vi "Breakdown Analysis Report.vi"(8 "error in (no error)":errorcluster) -> ()   [LabVIEW 2017]
uses:
  <vilib>/Utility/miscctls.llb/LVRowAndColumnTypeDef.ctl
  <vilib>/addons/database/Connection.llb/DB Tools Open Connec (Path).vi
  <vilib>/Utility/file.llb/Write Delimited Spreadsheet (string).vi
  <vilib>/addons/database/NI_Database_API.lvlib
panel:
  in  "Back 2":bool
  in  "Download 2":bool
  in  "Get Rport":bool
  out "index of element":i32
  out "Array":string[][](array[string])
  in  "(X,Y)":string
  out "subarray":string[](array[string])
  in  "Export to Excel":bool
  in  "Shift":string(combo)
  out "error out":errorcluster
  in  "Tab Control":enum32{"Statistical", "Graphical"}(tab)
  out "Table":string[][](table)
  out "Run-Time Status":cluster{dbl[], dbl[]}(graph)
  in  "Select Line":string(combo)
  in  "To Date":timestamp format="%<%Y-%m-%d>T"
  in  "Form Date":timestamp format="%<%Y-%m-%d>T"
  in  "Delete":bool
  in  "Edit":bool
  in  "Select Stakeholder":string(combo)
  in  "Get Report":bool
  # "Breakdown Analysis Report"
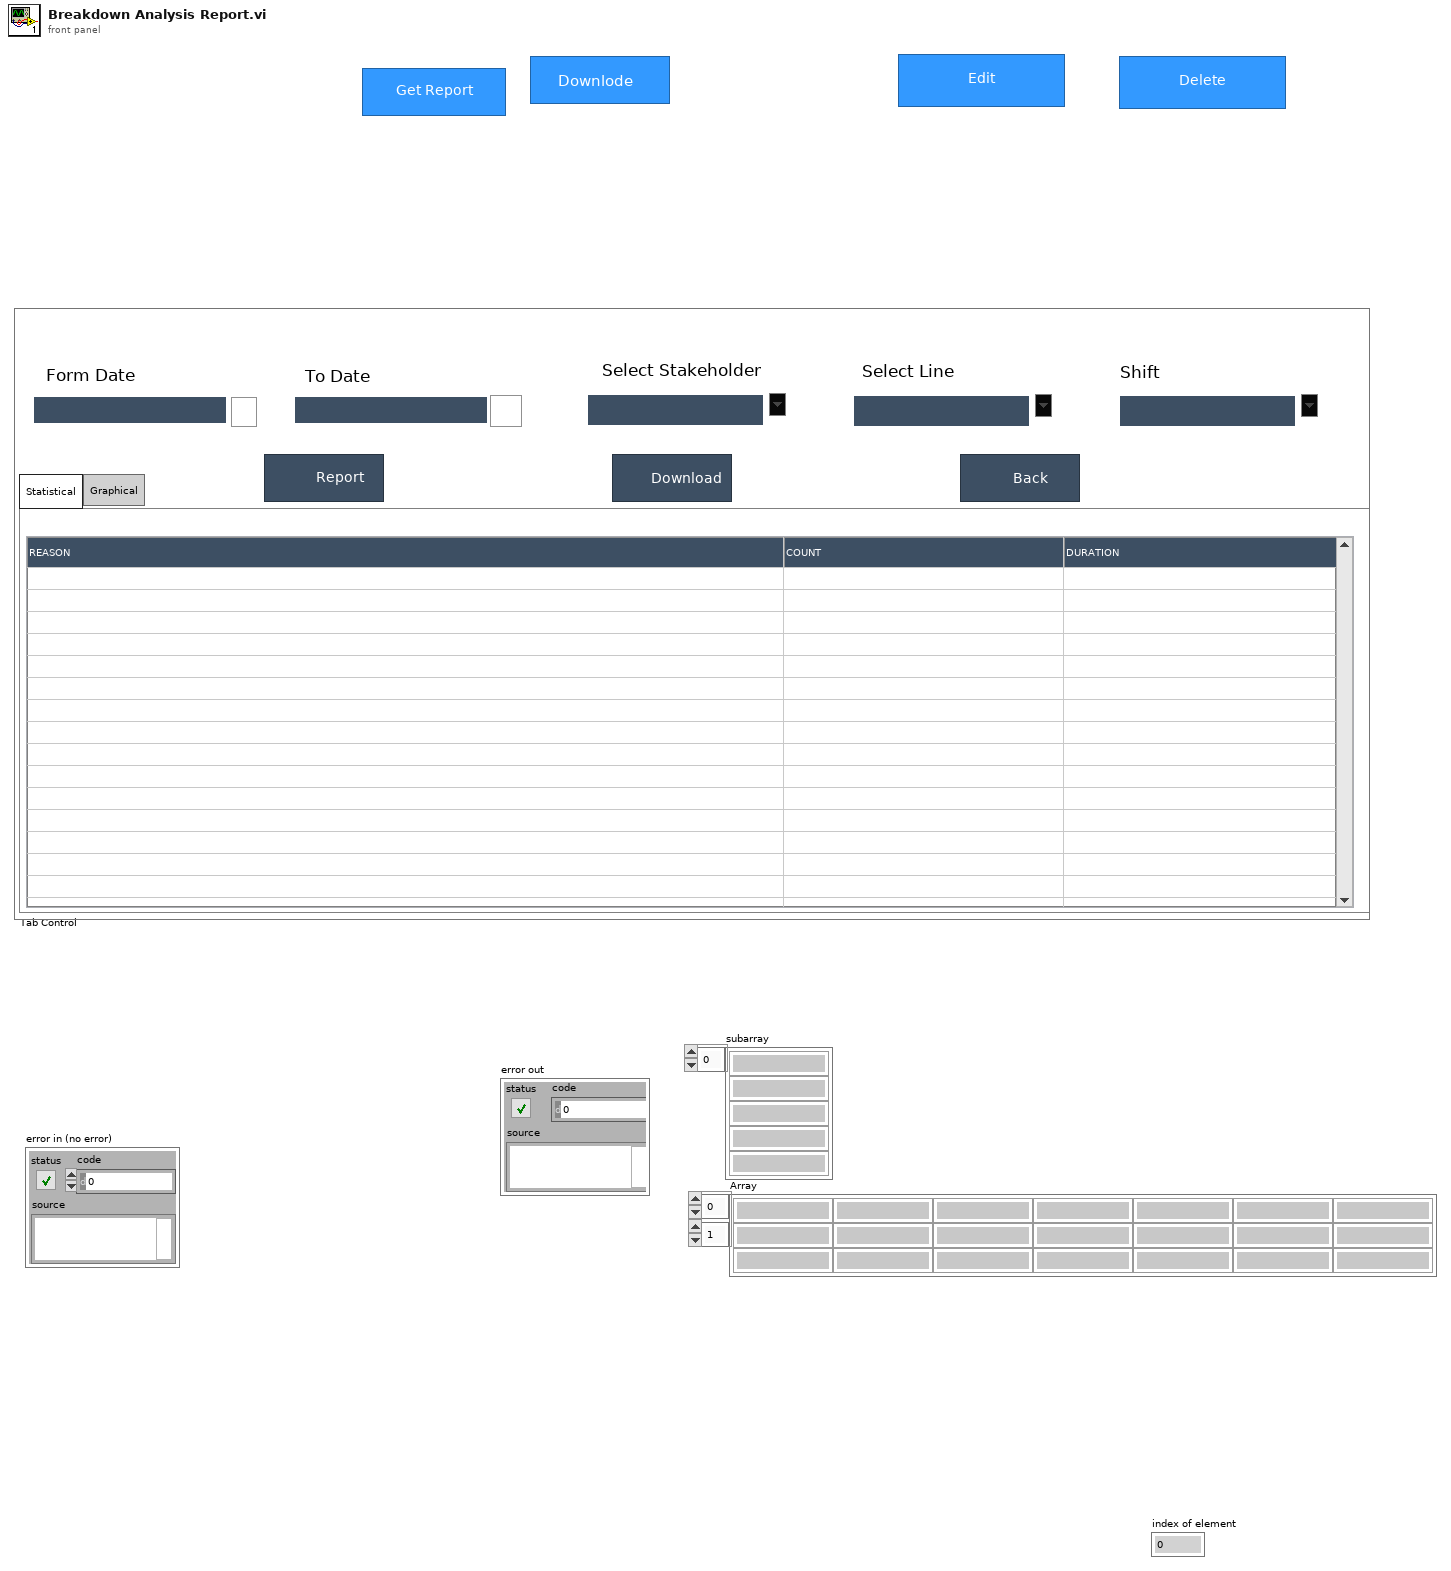
[diagram p1: front panel]
types:
  T1 = typedef "LVRowAndColumnTypeDef.ctl" = cluster{"Row":i32, "Column":i32}
  T2 = typedef "NI_Database_API.lvlib/Conn ObjectReference.ctl" = refnum<k1>
  T3 = typedef "LVPoint32TypeDef.ctl" = cluster{"Horizontal":i32, "Vertical":i32}
  T4 = enum32{"invalid app kind", "Development System", "Run Time System", "Student Edition", "Embedded LabVIEW", "Evaluation", "Custom"}
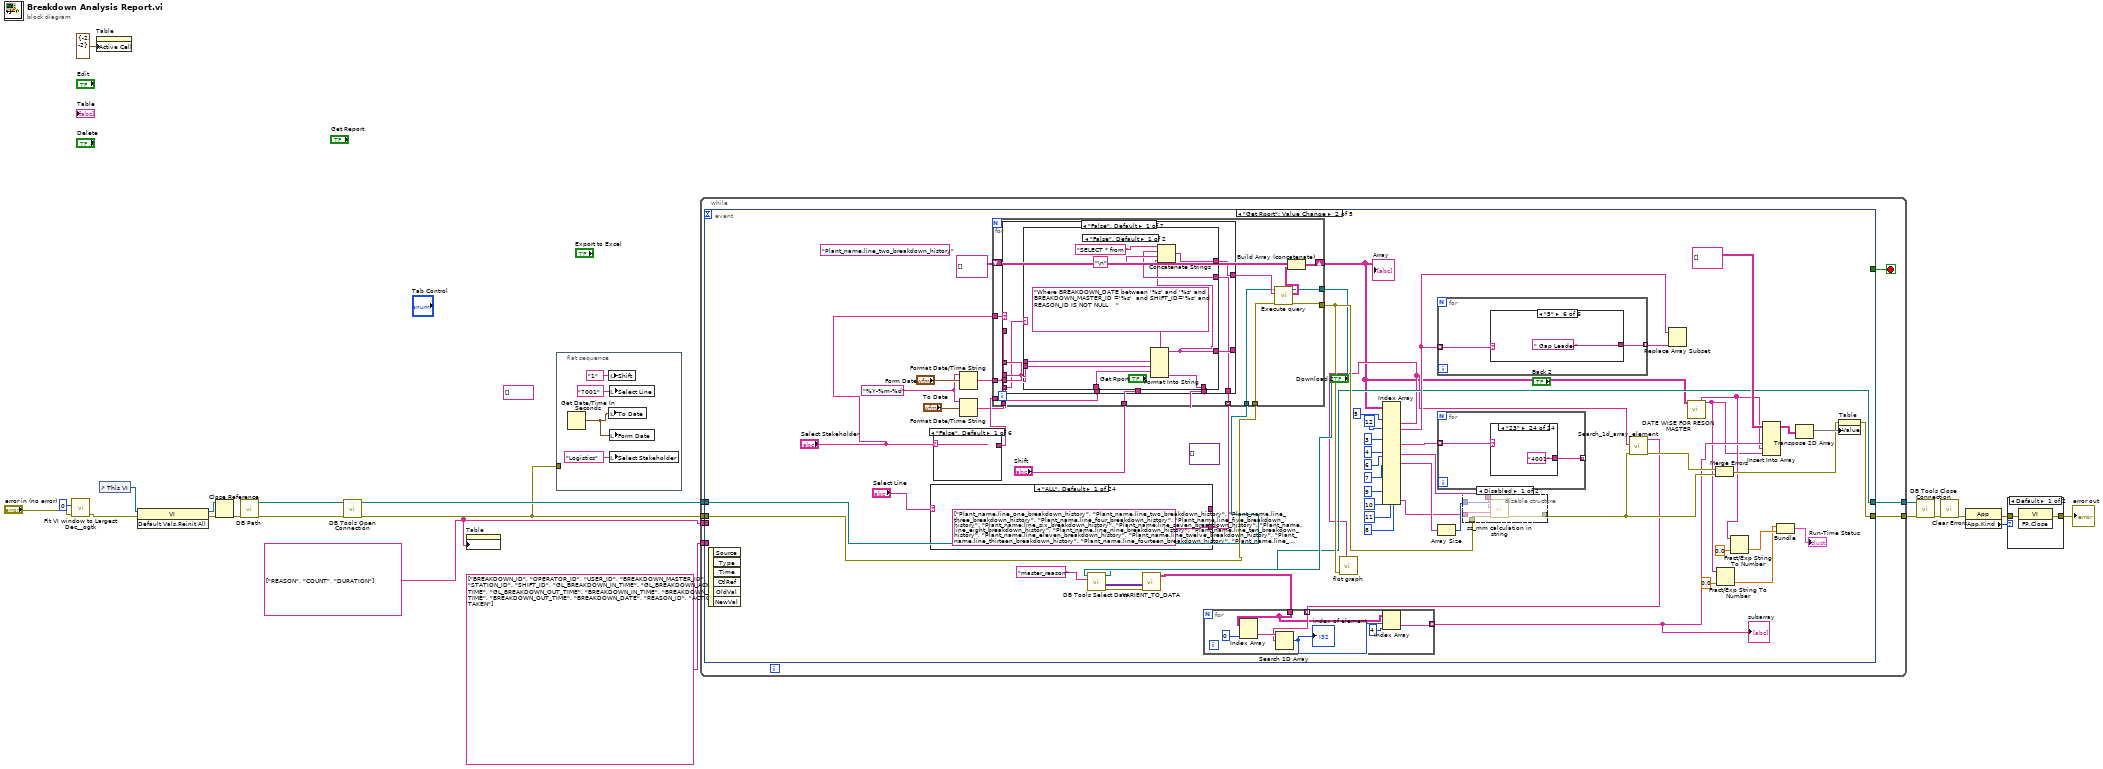
[diagram p0: block diagram]
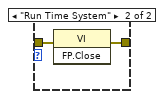
[diagram p2: hidden frame]
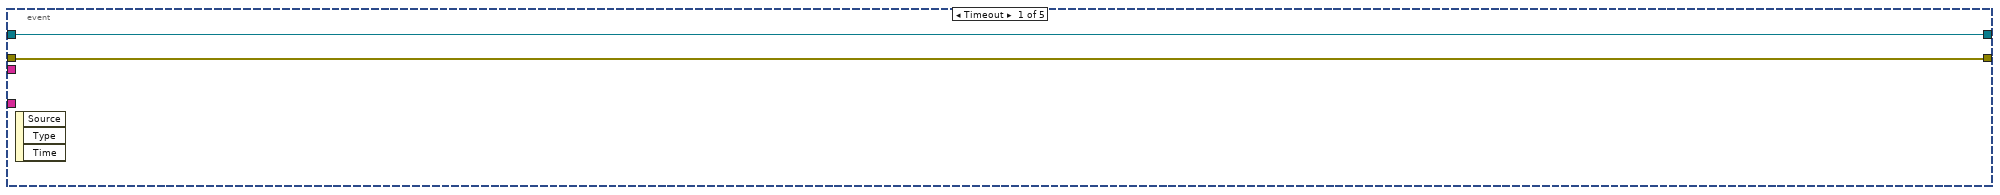
[diagram p3: hidden frame]
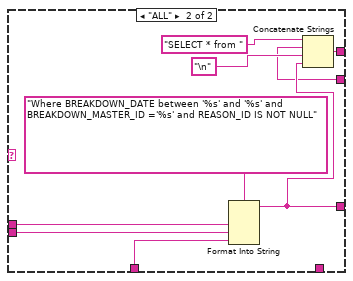
[diagram p5: hidden frame]
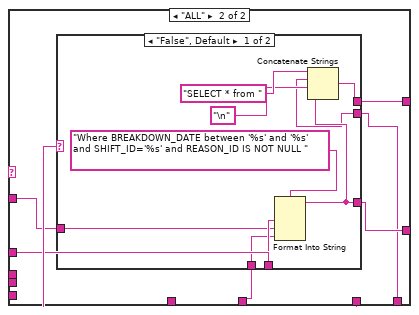
[diagram p6: hidden frame]
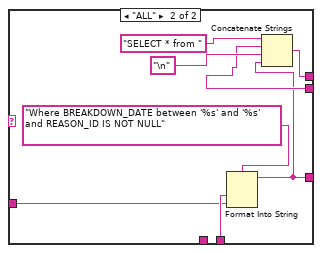
[diagram p7: hidden frame]
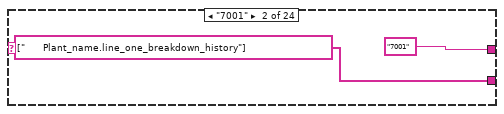
[diagram p8: hidden frame]
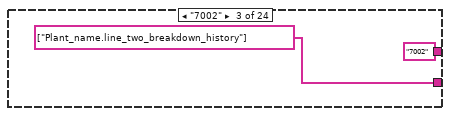
[diagram p9: hidden frame]
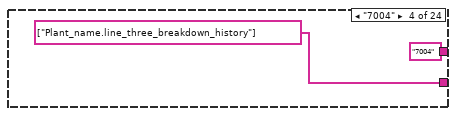
[diagram p10: hidden frame]
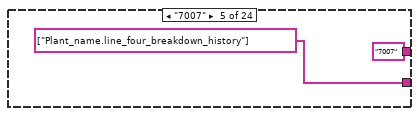
[diagram p11: hidden frame]
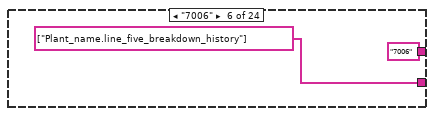
[diagram p12: hidden frame]
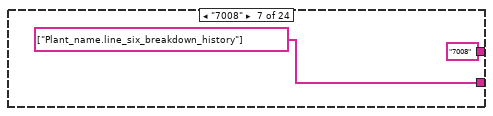
[diagram p13: hidden frame]
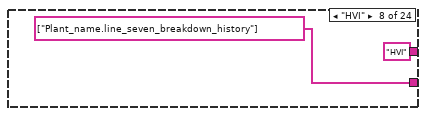
[diagram p14: hidden frame]
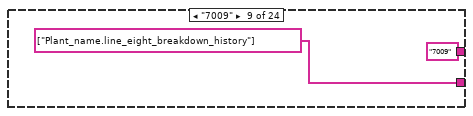
[diagram p15: hidden frame]
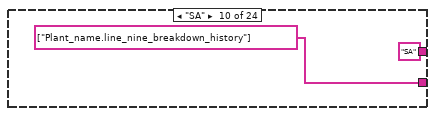
[diagram p16: hidden frame]
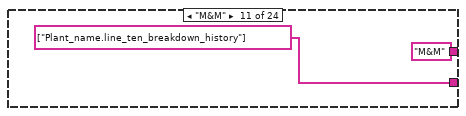
[diagram p17: hidden frame]
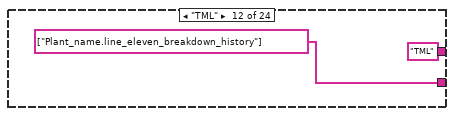
[diagram p18: hidden frame]
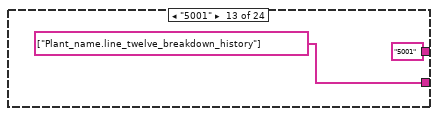
[diagram p19: hidden frame]
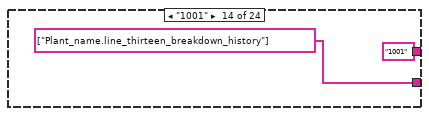
[diagram p20: hidden frame]
diagram:
  (unwired) string[] []
  w1 = string[] ["REASON", "COUNT", "DURATION"] ("Column Header Strings[]")
  n1 = call <userlib>:"Fit VI window to Largest Dec__ogtk.vi"("error in (no error)"="error in (no error)", "border spacing (2 px)"=0) -> ("error out"=w4:errorcluster)  [unwired: 4 in, 1 out]
  n2 = property on="Table" class="Tbl (strict)"("Active Cell"=T1 {"Row"=-2, "Column"=-2} ("Active Cell:Active Cell")) -> ()  [unwired: 2 in, 2 out]
  n3 = control-ref of="This VI"() -> (w20:refnum<vi>)
  n4 = invoke class="VI" method="Default Vals.Reinit All"(reference=w20, error in=w4) -> (reference out=w18:refnum<vi>, error out=w19:errorcluster)  [unwired: 1 in, 1 out]
  n5 = Close Reference(reference=w18, error in (no error)=w19) -> (error out=w11:errorcluster)
  n6 = call "DB Path.vi"("error in"=w11) -> ("error out"=w10:errorcluster, "DB Path"=w9:path)  [unwired: 9 in]
  n7 = call-poly <vilib>:"DB Tools Open Connection.vi"("error in (no error)"=w10, "connection information"=w9) -> ("error out"=w2:errorcluster, "connection reference"=w8:T2)  [unwired: 6 in]
  n8 = property on="Table" class="Tbl (strict)"("Column Headers[]"=w1) -> ()  [unwired: 2 in, 2 out]
  n9 = flat-sequence {
    tunnel: w2 -> [_]
    frame #0 {
      n10 = Get Date/Time In Seconds() -> (seconds since 1Jan1904=w25:timestamp)
      n11 = local write "Shift"("1" ("Shift")) -> ()
      n12 = local write "To Date"(w25) -> ()
      n13 = local write "Select Line"("7001" ("Select Line")) -> ()
      n14 = local write "Form Date"(w25) -> ()
      n15 = local write "Select Stakeholder"("Logistics" ("Select Stakeholder")) -> ()
    }
  }
  n16 = while {
    tunnel: w2 -> [w32]
    tunnel: [w31] -> w14
    tunnel: [w29] -> w12
    tunnel: w8 -> [w28]
    tunnel: string[] ["BREAKDOWN_ID", "OPERATOR_ID", "USER_ID", "BREAKDOWN_MASTER_ID", "STATION_ID", "SHIFT_ID", "GL_BREAKDOWN_IN_TIME", "GL_BREAKDOWN_ACK_TIME", "GL_BREAKDOWN_OUT_TIME", "BREAKDOWN_IN_TIME", "BREAKDOWN_ACK_TIME", "BREAKDOWN_OUT_TIME", "BREAKDOWN_DATE", "REASON_ID", "ACTION_TAKEN"] ("columns") -> [w27]
    tunnel: w1 -> [w26]
    stop <- w30 stop-if-true
    n17 = event shown="[1] \"Get Rport\": Value Change" {
      selector: _ -> [_ _ _ _ _]
      dyn-events: _ -> [_ _ _ _ _]
      timeout: _ -> [_ _ _ _ _]
      tunnel: w32 -> [w34 w59 _ w273 _]
      tunnel: [w34 w67 _ w268 _] -> w31
      tunnel: [_ _ _ _ TRUE] -> w30
      tunnel: [w33 w50 _ _ _] -> w29
      tunnel: w28 -> [w33 w53 _ _ _]
      tunnel: w27 -> [_ _ _ _ _]
      tunnel: w26 -> [_ _ _ _ _]
      event Timeout {
        n18 = event-data() -> ()  [unwired: 1 in, 3 out]
      }
      event "Get Rport": Value Change {
        (unwired) variant[][] [] ("data")
        (unwired) "Plant_name.line_two_breakdown_history" ("table")
        w86 = "%Y-%m-%d" ("time format string (%c)")
        n19 = event-data() -> ()  [unwired: 1 in, 6 out]
        n20 = case shown="\"ALL\", Default" "Select Line" {
          tunnel: [_ "7001" "7002" "7004" "7007" "7006" "7008" "HVI" "7009" "SA" "M&M" "TML" "5001" "1001" "4003" "1002" "4004" "1004" "2001" "3001" "2004" "3002" "3003" "4001"] -> _
          tunnel: [string[] ["Plant_name.line_one_breakdown_history", "Plant_name.line_two_breakdown_history", "Plant_name.line_three_breakdown_history", "Plant_name.line_four_breakdown_history", "Plant_name.line_five_breakdown_history", "Plant_name.line_six_breakdown_history", "Plant_name.line_seven_breakdown_history", "Plant_name.line_eight_breakdown_history", "Plant_name.line_nine_breakdown_history", "Plant_name.line_ten_breakdown_history", "Plant_name.line_eleven_breakdown_history", "Plant_name.line_twelve_breakdown_history", "Plant_name.line_thirteen_breakdown_history", "Plant_name.line_fourteen_breakdown_history", "Plant_name.line_fifteen_breakdown_history", "Plant_name.line_sixteen_breakdown_history", "Plant_name.line_seventeen_breakdown_history", "Plant_name.line_eighteen_breakdown_history", "Plant_name.line_nineteen_breakdown_history", "Plant_name.line_twenty_breakdown_history", "Plant_name.line_twenty_one_breakdown_history", "Plant_name.line_twenty_two_breakdown_history", "Plant_name.line_twenty_three_breakdown_history"] string[] ["      Plant_name.line_one_breakdown_history"] string[] ["Plant_name.line_two_breakdown_history"] string[] ["Plant_name.line_three_breakdown_history"] string[] ["Plant_name.line_four_breakdown_history"] string[] ["Plant_name.line_five_breakdown_history"] string[] ["Plant_name.line_six_breakdown_history"] string[] ["Plant_name.line_seven_breakdown_history"] string[] ["Plant_name.line_eight_breakdown_history"] string[] ["Plant_name.line_nine_breakdown_history"] string[] ["Plant_name.line_ten_breakdown_history"] string[] ["Plant_name.line_eleven_breakdown_history"] string[] ["Plant_name.line_twelve_breakdown_history"] string[] ["Plant_name.line_thirteen_breakdown_history"] string[] ["Plant_name.line_fourteen_breakdown_history"] string[] ["Plant_name.line_fifteen_breakdown_history"] string[] ["Plant_name.line_sixteen_breakdown_history"] string[] ["Plant_name.line_seventeen_breakdown_history"] string[] ["Plant_name.line_eighteen_breakdown_history"] string[] ["Plant_name.line_nineteen_breakdown_history"] string[] ["Plant_name.line_twenty_breakdown_history"] string[] ["Plant_name.line_twenty_one_breakdown_history"] string[] ["Plant_name.line_twenty_two_breakdown_history"] string[] ["Plant_name.line_twenty_three_breakdown_history"]] -> w58
          frame "ALL", Default {
          }
          frame "7001" {
          }
          frame "7002" {
          }
          frame "7004" {
          }
          frame "7007" {
          }
          frame "7006" {
          }
          frame "7008" {
          }
          frame "HVI" {
          }
          frame "7009" {
          }
          frame "SA" {
          }
          frame "M&M" {
          }
          frame "TML" {
          }
          frame "5001" {
          }
          frame "1001" {
          }
          frame "4003" {
          }
          frame "1002" {
          }
          frame "4004" {
          }
          frame "1004" {
          }
          frame "2001" {
          }
          frame "3001" {
          }
          frame "2004" {
          }
          frame "3002" {
          }
          frame "3003" {
          }
          frame "4001" {
          }
        }
        n21 = case shown="\"False\", Default" "Select Stakeholder" {
          tunnel: [_ "1" "2" "3" "4" "5"] -> w87
          frame "False", Default {
          }
          frame "Logistics" {
          }
          frame "Maintenance" {
          }
          frame "Quality" {
          }
          frame "Production" {
          }
          frame "Gap Leader" {
          }
        }
        n22 = Format Date/Time String(time format string (%c)=w86, seconds (now)="Form Date") -> (date/time string=w64:string)  [unwired: 1 in]
        n23 = Format Date/Time String(time format string (%c)=w86, seconds (now)="To Date") -> (date/time string=w63:string)  [unwired: 1 in]
        n24 = for {
          tunnel: "Select Stakeholder" -> [w114]
          tunnel: w64 -> [w113]
          tunnel: w63 -> [w112]
          tunnel: "Shift" -> [w111]
          tunnel: w87 -> [w115]
          tunnel: w58 -> [w110] mode=indexing
          shift-right: [w107] -> w43
          shift-left: string[][] [] -> [w106]
          tunnel: w59 -> [w105]
          tunnel: [w104] -> w57
          tunnel: w53 -> [w103]
          tunnel: [w102] -> w51
          n25 = case shown="\"False\", Default" w114 {
            tunnel: [w118 w145] -> _
            tunnel: w113 -> [w123 _]
            tunnel: w112 -> [w122 _]
            tunnel: w115 -> [w121 _]
            tunnel: w111 -> [w120 w149]
            tunnel: w111 -> [w119 _]
            tunnel: w113 -> [_ w148]
            tunnel: w112 -> [_ w147]
            tunnel: w111 -> [_ w146]
            tunnel: w110 -> [w117 w143]
            tunnel: [w116 w144] -> w109
            frame "False", Default {
              n26 = case shown="\"False\", Default" w119 {
                tunnel: [w124 w136] -> w118
                tunnel: w123 -> [w132 w141]
                tunnel: w122 -> [w131 w140]
                tunnel: w121 -> [w130 w139]
                tunnel: w120 -> [w129 _]
                tunnel: w117 -> [w125 w135]
                tunnel: [w126 w134] -> w116
                frame "False", Default {
                  n27 = Format Into String(format string="Where BREAKDOWN_DATE between '%s' and '%s' and BREAKDOWN_MASTER_ID ='%s'  and SHIFT_ID='%s' and REASON_ID IS NOT NULL    " ("condition"), w132, w131, w130, w129) -> (resulting string=w124:string)  [unwired: 2 in, 1 out]
                  n28 = Concatenate Strings("SELECT * from " ("String"), w125, "\n" ("string"), w124) -> (w126:string)
                }
                frame "ALL" {
                  n29 = Format Into String(format string="Where BREAKDOWN_DATE between '%s' and '%s' and BREAKDOWN_MASTER_ID ='%s' and REASON_ID IS NOT NULL" ("condition"), w141, w140, w139) -> (resulting string=w136:string)  [unwired: 2 in, 1 out]
                  n30 = Concatenate Strings("SELECT * from " ("String"), w135, "\n" ("string"), w136) -> (w134:string)
                }
              }
            }
            frame "ALL" {
              n31 = case shown="\"False\", Default" w149 {
                tunnel: w148 -> [w158 w165]
                tunnel: w147 -> [w157 w164]
                tunnel: w146 -> [w156 _]
                tunnel: [w151 w160] -> w145
                tunnel: [w152 w159] -> w144
                tunnel: w143 -> [w150 w162]
                frame "False", Default {
                  n32 = Format Into String(format string="Where BREAKDOWN_DATE between '%s' and '%s' and SHIFT_ID='%s' and REASON_ID IS NOT NULL " ("condition"), w158, w157, w156) -> (resulting string=w151:string)  [unwired: 2 in, 1 out]
                  n33 = Concatenate Strings("SELECT * from " ("String"), w150, "\n" ("string"), w151) -> (w152:string)
                }
                frame "ALL" {
                  n34 = Format Into String(format string="Where BREAKDOWN_DATE between '%s' and '%s' and REASON_ID IS NOT NULL" ("condition"), w165, w164) -> (resulting string=w160:string)  [unwired: 2 in, 1 out]
                  n35 = Concatenate Strings("SELECT * from " ("String"), w162, "\n" ("string"), w160) -> (w159:string)
                }
              }
            }
          }
          n36 = call "Execute query.vi"("error in (no error)"=w105, "String"=w109, "connection reference"=w103) -> ("error out"=w104:errorcluster, "Table"=w108:string[][], "connection reference 2"=w102:T2)  [unwired: 5 in, 1 out]
          n37 = Build Array (concatenate)(w106, w108) -> (w107:string[][])
        }
        "Array" <- w43
        n38 = call <vilib>:"DB Tools Select Data.vi"("table"="master_reason", "connection reference"=w51) -> ("error out"=w56:errorcluster, "data"=w55:variant[][], "connection reference out"=w50:T2)  [unwired: 4 in]
        n39 = call "VARIENT_TO_DATA.vi"("data"=w55, "error in (no error)"=w56) -> ("Table"=w54:string[][])  [unwired: 7 in, 1 out]
        n40 = Index Array(array=w43, index (col) #1=5 ("disabled index (col)"), index (col) #2=12 ("disabled index (col)"), index (col) #3=3 ("index (col)"), index (col) #4=4 ("index (col)"), index (col) #5=6 ("index (col)"), index (col) #6=7 ("index (col)"), index (col) #7=9 ("index (col)"), index (col) #8=10 ("index (col)"), index (col) #9=11 ("index (col)"), index (col) #10=8 ("index (col)")) -> (element #2=w49:string[], element #3=w83:string[], element #4=w71:string[], element #5=w68:string[], element #6=w70:string[], element #10=w35:string[])  [unwired: 10 in, 4 out]
        n41 = call "flot graph.vi"("BD Date"=w49, "error in (no error)"=w57) -> ()  [unwired: 9 in, 1 out]
        n42 = for {
          tunnel: w83 -> [w240] mode=indexing
          tunnel: [w239] -> w82 mode=indexing
          n43 = case shown="\"5\"" w240 {
            tunnel: ["all" "Logistics" "Maintenance" "Quality" "Production" " Gap Leader"] -> w239
            frame "False", Default {
            }
            frame "1" {
            }
            frame "2" {
            }
            frame "3" {
            }
            frame "4" {
            }
            frame "5" {
            }
          }
        }
        n44 = for {
          tunnel: w71 -> [w215] mode=indexing
          tunnel: [w214] -> _ mode=indexing
          n45 = case shown="\"23\"" w215 {
            tunnel: [_ "7001" "7002" "7004" "7007" "7006" "7008" "HVI" "7009" "SA" "M&M" "TML" "5001" "1001" "4003" "1002" "4004" "1004" "2001" "3001" "2004" "3002" "3003" "4001"] -> w214
            frame "0", Default {
            }
            frame "1" {
            }
            frame "2" {
            }
            frame "3" {
            }
            frame "4" {
            }
            frame "5" {
            }
            frame "6" {
            }
            frame "7" {
            }
            frame "8" {
            }
            frame "9" {
            }
            frame "10" {
            }
            frame "11" {
            }
            frame "12" {
            }
            frame "13" {
            }
            frame "14" {
            }
            frame "15" {
            }
            frame "16" {
            }
            frame "17" {
            }
            frame "18" {
            }
            frame "19" {
            }
            frame "20" {
            }
            frame "21" {
            }
            frame "22" {
            }
            frame "23" {
            }
          }
        }
        n46 = Array Size(array=w70) -> (size(s)=w69:i32)
        n47 = disable-structure shown="Disabled" {
          disable-tunnel: w69 -> [w94 _]
          disable-tunnel: w35 -> [w93 _]
          disable-tunnel: w68 -> [w92 _]
          disable-tunnel: w57 -> [w91 _]
          disable-tunnel: [w90 _] -> w47
          frame Disabled {
            n48 = call "ss_mm calculation in string.vi"("error in (no error)"=w91, "Table 2"=w93, "Table"=w92, "Numeric"=w94) -> ("error out"=w90:errorcluster)  [unwired: 6 in, 1 out]
          }
          frame Enabled {
          }
        }
        n49 = call "Search_1d_array_element.vi"("error in (no error)"=w47, "BD Date"=w49) -> ("error out"=w48:errorcluster, "Elements Found out"=w45:string[])  [unwired: 5 in, 1 out]
        n50 = for {
          tunnel: w54 -> [w95]
          tunnel: w45 -> [w97] mode=indexing
          tunnel: [w96] -> w44 mode=indexing
          n51 = Index Array(array=w95, index (col)=0 ("disabled index (col)")) -> (element=w100:string[])  [unwired: 1 in]
          n52 = Search 1D Array(1D array=w100, element=w97) -> (index of element=w101:i32)  [unwired: 1 in]
          "index of element" <- w101
          n53 = Index Array(array=w95, index (row)=w101, index (col)=4 ("disabled index (col)")) -> (element=w96:string)
        }
        "subarray" <- w44
        n54 = Replace Array Subset(array=w83, new element=w82) -> ()  [unwired: 1 in, 1 out]
        n55 = call "DATE WISE FOR RESON MASTER.vi"("Array"=w43) -> ("Count out"=w42:string[], "DURATION"=w41:string[])  [unwired: 12 in, 5 out]
        n56 = Merge Errors(w48, w47) -> (w46:errorcluster)
        n57 = Fract/Exp String To Number(string=w41, default (0 dbl)=0.0 ("default (0 DBL)")) -> (number=w36:dbl[])  [unwired: 2 in, 1 out]
        n58 = Fract/Exp String To Number(string=w42, default (0 dbl)=0.0 ("default (0 DBL)")) -> (number=w38:dbl[])  [unwired: 2 in, 1 out]
        n59 = Insert Into Array(array=string[][] [], new element #1=w44, new element #2=w42, new element #3=w41) -> (w80:string[][])  [unwired: 2 in]
        n60 = Bundle(w36, w38) -> (→"Run-Time Status":cluster{dbl[], dbl[]})  [unwired: 1 in]
        n61 = Transpose 2D Array(2D array=w80) -> (transposed array=w79:string[][])
        n62 = property on="Table" class="Tbl (strict)"(error in=w46, "Value"=w79) -> (error out=w67:errorcluster)  [unwired: 1 in, 1 out]
      }
      event "Run-Time Status": Mouse Move {
        # "Display the coordinate in \nthe string indicator"
        # "Get XY value of the graph"
        # "When mouse are not at graph curve, \nreturn value as -1"
        # "Check whether mouse on graph curve"
        n63 = event-data() -> ("Coords"=w255:T3)  [unwired: 1 in, 4 out]
        n64 = control-ref of="Run-Time Status"() -> (w254:refnum<vi>)
        n65 = invoke on="Invoke Node" class="XYGraph (strict)" method="GetPlotAtPos"(reference=w254, "InputPt"=w255) -> ("PlotNum"=w260:i32)  [unwired: 3 in, 4 out]
        n66 = invoke on="Invoke Node" class="XYGraph (strict)" method="Map Coords To XY"(reference=w254, "Coords"=w255) -> ("XY"=w267:cluster{"X":dbl, "Y":dbl})  [unwired: 5 in, 6 out]
        n67 = Not Equal?(x=-1, y=w260) -> (x != y?=w258:bool)
        n68 = Unbundle(w267) -> ("X"=w253:dbl, "Y"=w266:dbl)
        n69 = Number To Fractional String(number=w266, precision (6)=i16 0) -> (F-format string=w263:string)  [unwired: 2 in]
        n70 = Number To Fractional String(number=w253) -> (F-format string=w252:string)  [unwired: 3 in]
        n71 = control-ref of="(X,Y)"() -> (w256:refnum<vi>)
        n72 = Concatenate Strings("(" ("string"), w252, "," ("string"), w263, ")" ("string")) -> (w257:string)
        n73 = property on="Property Node" class="Str"(reference=w256, "Visible"=w258, "Position"=w255, "Value"=w257) -> ()  [unwired: 1 in, 2 out]
      }
      event "Download 2": Value Change {
        n74 = event-data() -> ()  [unwired: 1 in, 6 out]
        n75 = call "File Dialog"() -> ("selected path"=w277:path, "error out"=w276:errorcluster)  [unwired: 12 in, 2 out]
        n76 = call <vilib>:"Clear Errors.vi"("error in (no error)"=w276) -> ()  [unwired: 5 in, 2 out]
        n77 = Path To String(path=w277) -> (string=w278:string)
        n78 = Concatenate Strings(w278, ".csv" ("string")) -> (w279:string)
        n79 = property on="Table" class="Tbl (strict)"() -> ("Value"=w274:string[][])  [unwired: 2 in, 2 out]
        n80 = String To Path(string=w279) -> (path=w280:path)
        n81 = Build Array (concatenate)(string[][] [["Reason", "Count", "Duration"]] ("Column Header Strings[]"), w274) -> (w270:string[][])
        n82 = call-poly <vilib>:"Write Delimited Spreadsheet.vi"("file path (dialog if empty)"=w280, "2D data"=w270, "error in (no error)"=w273, "delimiter (\\t)"="," ("delimiter (\\t)")) -> ("error out"=w269:errorcluster)  [unwired: 10 in, 1 out]
        n83 = call <vilib>:"Clear Errors.vi"("error in (no error)"=w269) -> ("error out"=w268:errorcluster)  [unwired: 5 in, 1 out]
      }
      event "Back 2": Value Change {
        n84 = event-data() -> ()  [unwired: 1 in, 6 out]
      }
    }
  }
  n85 = call <vilib>:"DB Tools Close Connection.vi"("error in (no error)"=w14, "connection reference"=w12) -> ("error out"=w15:errorcluster)  [unwired: 5 in]
  n86 = call <vilib>:"Clear Errors.vi"("error in (no error)"=w15) -> ("error out"=w13:errorcluster)  [unwired: 5 in, 1 out]
  n87 = property class="App"(error in=w13) -> (error out=w16:errorcluster, "App.Kind"=w17:T4)  [unwired: 1 in, 1 out]
  n88 = case shown="Default" w17 {
    tunnel: w16 -> [w283 w285]
    tunnel: [w282 w284] -> w6
    frame Default {
      n89 = invoke class="VI" method="FP.Close"(error in=w283) -> (error out=w282:errorcluster)  [unwired: 2 in, 2 out]
    }
    frame "Run Time System" {
      n90 = invoke class="VI" method="FP.Close"(error in=w285) -> (error out=w284:errorcluster)  [unwired: 2 in, 2 out]
    }
  }
  "error out" <- w6
